vi "Chord to Center.vi"(11 "Tag points":T1) -> (1 "output circle info":T2, 2 "T2 endPt":cluster{dbl, dbl}, 3 "T1 endPt":cluster{dbl, dbl}, 4 "angle T1 to T2":dbl)   [LabVIEW 2025]
panel:
  in  "stroke length":dbl=10.0 format="%#_13g"
  out "delta angle":dbl
  out "length of chord":dbl
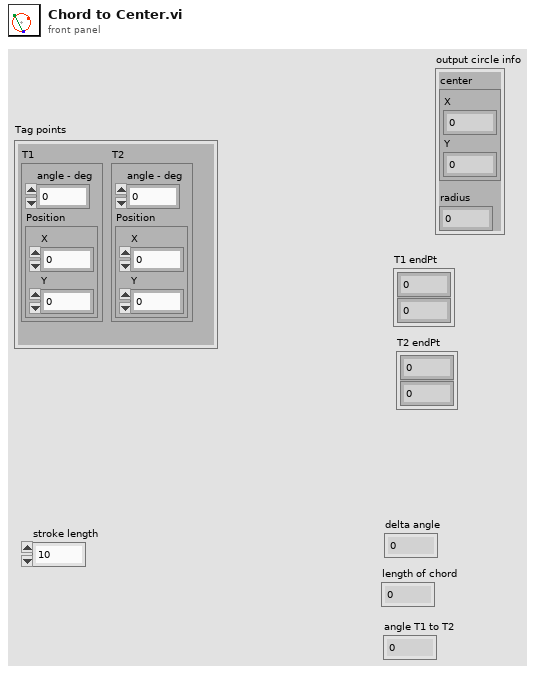
[diagram p1: front panel]
types:
  T1 = cluster{"T1":cluster{"angle - deg":dbl, "Position":cluster{"X":dbl, "Y":dbl}}, "T2":cluster{"angle - deg":dbl, "Position":cluster{"X":dbl, "Y":dbl}}}
  T2 = cluster{"center":cluster{"X":sgl, "Y":sgl}, "radius":sgl}
  T3 = cluster{"angle - deg":dbl, "Position":cluster{"X":dbl, "Y":dbl}}
  T4 = cluster{"Position":cluster{"X":dbl, "Y":dbl}, cluster{dbl, dbl}}
  T5 = cluster{"Intersection Point":cluster{"X":sgl, "Y":sgl}, sgl}
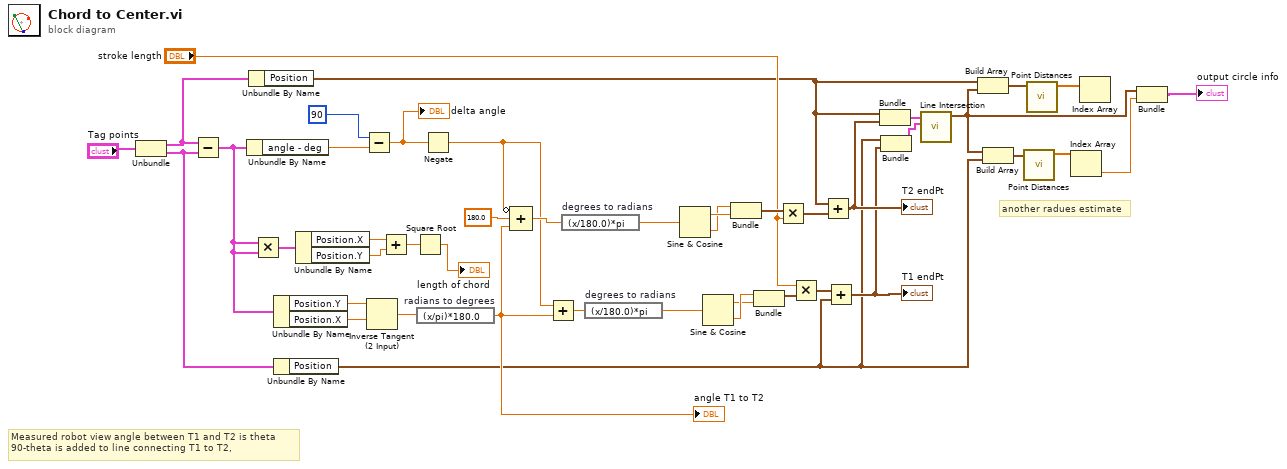
[diagram p0: block diagram]
diagram:
  # "another radues estimate"
  # "Measured robot view angle between T1 and T2 is theta\n90-theta is added to line connecting T1 to T2,"
  n1 = Unbundle("Tag points") -> ("T1"=w6:T3, "T2"=w5:T3)
  n2 = Subtract(x=w6, y=w5) -> (x-y=w32:T3)
  n3 = Unbundle By Name(w32) -> ("angle - deg"=w3:dbl)
  n4 = Unbundle By Name(w6) -> ("Position"=w15:cluster{"X":dbl, "Y":dbl})
  n5 = Multiply(x=w32, y=w32) -> (x*y=w28:T3)
  n6 = Unbundle By Name(w32) -> ("Position.Y"=w33:dbl, "Position.X"=w34:dbl)
  n7 = Unbundle By Name(w5) -> ("Position"=w13:cluster{"X":dbl, "Y":dbl})
  n8 = Unbundle By Name(w28) -> ("Position.X"=w29:dbl, "Position.Y"=w30:dbl)
  n9 = Subtract(x=90, y=w3) -> (x-y=w2:dbl)
  "delta angle" <- w2
  n10 = Inverse Tangent (2 Input)(1:w34, 2:w33) -> (0:w35:dbl)
  n11 = Add(x=w29, y=w30) -> (x+y=w31:dbl)
  n12 = Square Root(x=w31) -> (sqrt(x)=→"length of chord":dbl)
  n13 = expression code="(x/pi)*180.0" "radians to degrees"(w35) -> (w43:dbl)
  "angle T1 to T2" <- w43
  n14 = Negate(x=w2) -> (-x=w1:dbl)
  n15 = Compound Arithmetic op=ADD(invert w1, 180.0 ("x"), w43) -> (w23:dbl)
  n16 = Add(x=w1, y=w43) -> (x+y=w41:dbl)
  n17 = expression code="(x/180.0)*pi" "degrees to radians"(w23) -> (w24:dbl)
  n18 = expression code="(x/180.0)*pi" "degrees to radians"(w41) -> (w42:dbl)
  n19 = Sine & Cosine(0:w24) -> (1:w26:dbl, 2:w25:dbl)
  n20 = Sine & Cosine(0:w42) -> (1:w36:dbl, 2:w37:dbl)
  n21 = Bundle(w25, w26) -> (w22:cluster{dbl, dbl})  [unwired: 1 in]
  n22 = Bundle(w37, w36) -> (w38:cluster{dbl, dbl})  [unwired: 1 in]
  n23 = Multiply(x=w22, y="stroke length") -> (x*y=w20:cluster{dbl, dbl})
  n24 = Multiply(x="stroke length", y=w38) -> (x*y=w40:cluster{dbl, dbl})
  n25 = Add(x=w15, y=w20) -> (x+y=w19:cluster{dbl, dbl})
  "T2 endPt" <- w19
  n26 = Add(x=w40, y=w13) -> (x+y=w17:cluster{dbl, dbl})
  "T1 endPt" <- w17
  n27 = Bundle("Position"=w15, w19) -> (w18:T4)  [unwired: 1 in]
  n28 = Bundle("Position"=w13, w17) -> (w16:T4)  [unwired: 1 in]
  n29 = call "Line Intersection.vi"("Line 2"=w16, "Line 1"=w18) -> ("Intersection Point"=w9:cluster{"X":sgl, "Y":sgl})  [unwired: 9 in]
  n30 = Build Array(w15, w9) -> (w14:cluster{"X":dbl, "Y":dbl}[])
  n31 = Build Array(w9, w13) -> (w12:cluster{"X":dbl, "Y":dbl}[])
  n32 = call "Point Distances.vi"("Points"=w12) -> ("Distances"=w10:sgl[])  [unwired: 10 in]
  n33 = call "Point Distances.vi"("Points"=w14) -> ("Distances"=w11:sgl[])  [unwired: 10 in]
  n34 = Index Array(array=w10) -> (element=w4:sgl)  [unwired: 1 in]
  n35 = Index Array(array=w11) -> ()  [unwired: 1 in, 1 out]
  n36 = Bundle("Intersection Point"=w9, w4) -> (→"output circle info":T5)  [unwired: 1 in]
